vi "DDS Only.vi"() -> ()   [LabVIEW 2013]
doc: "This is the main code used to run experiments in the Cesium laboratory of Mark Saffman. It was written by Martin Lichtman from 2009 to 2012, with DDS drivers written by Alex Gill and Larry Isenhower.\n\nEach hardware section may be enabled and disabled separately. Experiments will finish when all hardware has completed, or when the \"experiment timeout\" is reached, whichever comes first."
uses:
  ExperimentVariables/Variable_Settings.ctl
  DDS_Settings_Cluster.ctl
  DDS Library/Controls/DDS Box Array.ctl
  DDS Library/Controls/DDS Box Cluster.ctl
  DDS Library/Controls/DDS Box Device Reference.ctl
  <vilib>/ni845x/ni845x.llb/ni845xControl.ctl
  DDS Library/Controls/DDS Channel Array.ctl
  DDS Library/Controls/DDS Channel.ctl
  DDS Library/Controls/DDS Channel Parameters.ctl
  DDS Library/Controls/DDS RAM Destination.ctl
  DDS Library/Controls/DDS Profile Array.ctl
  DDS Library/Controls/DDS Profile.ctl
  DDS Library/Controls/DDS RAM Mode.ctl
  DDS Library/Controls/DDS RAM Timestep.ctl
  <vilib>/Utility/error.llb/DialogType.ctl
  config_file_io/all_settings.ctl
  HSDIO/HSDIO_settings.ctl
  <instrlib>/niHSDIO/niHSDIO.llb/niHSDIO_ctl Trigger Script - trigID Values (Ring).ctl
  <instrlib>/niHSDIO/niHSDIO.llb/niHSDIO_ctl Trigger Source Values (Ring).ctl
  <instrlib>/niHSDIO/niHSDIO.llb/niHSDIO_ctl Trigger DigEdge - Edge Values (Ring).ctl
  <instrlib>/niHSDIO/niHSDIO.llb/niHSDIO_ctl Trigger DigLvl - Level Values (Ring).ctl
  DAQmx_pulse_out/settings.ctl
  Camera/Hamamatsu_C9100-13/camera_setup.ctl
  Counter/Counter_Settings_Control.ctl
  filters/filters.ctl
  Analog_output/AO_settings.ctl
  GPIB/HP83623A_RF_Generator/HP83623A_settings.ctl
  PI_piezo/settings.ctl
  PI_piezo/PI_piezo_controller.ctl
  PI_piezo/PI_piezo_channel.ctl
  Camera/Andor/Andor_settings.ctl
  gui/measurement_graph.ctl
  GPIB/RF_Generator_settings_array.ctl
  GPIB/RF_Generator_settings.ctl
  TTL_input/TTL_input_settings.ctl
  Camera/Andor_Luca/Luca_Settings.ctl
  Camera/Andor_Luca/Acquisition_Mode.ctl
  Camera/Andor_Luca/Gain_Mode.ctl
  Aerotech/Aerotech_Settings.ctl
  CONEX-CC/Conex-CC Settings.ctl
  <vilib>/Utility/file.llb/Read From Spreadsheet File (string).vi
  GPIB/HP8662A_RF_Generator/HP8662A_RF_Generator.lvclass
  Camera/Andor_Luca/Andor_Luca.lvclass
  TTL_input/TTL_input.lvclass
  GPIB/GPIB.lvclass
  GPIB/HP83623A_RF_Generator/HP83623A_RF_Generator.lvclass
  Analog_output/Analog_Output.lvclass
  Counter/Counter.lvclass
  Camera/Hamamatsu_C9100-13/Hamamatsu_C9100-13.lvclass
  DDS Library/DDS.lvlib
  DAQmx_pulse_out/DAQmx_pulse_out.lvclass
  HSDIO/HSDIO.lvclass
  ExperimentVariables/ExperimentVariables.lvclass
  Aerotech/Aerotech.lvclass
  CONEX-CC/CONEX-CC.lvclass
panel:
  in  "Save Settings":bool
  in  "Load Settings":bool
  in  "Quit Program":bool=TRUE
  in  "Tab Control":enum32{"Experiment Variables", "DDS"}(tab)=enum."DDS"
  in  "Variable Actions":T1
  in  "Variable Settings":T2={"Measurements per Iteration"=5, "Local Data Path"=path "D:/Hybrid Experiment/Data", "Experiment description suffix for filename (no spaces please)"="TOF_SingleStage", "Network Data Path"=path "Z:/Public/Hybrid/Data/Measurements", "Copy data to network"=TRUE, "Measurement Timeout (ms)"=60000, "Independent Variables"=[{"Description"="MOT Load", "Name (a,a0...a9)"="m", "min"=2000.0, "max"=3000.0, "# steps"=1}, {"Description"="PGC Duration", "Name (a,a0...a9)"="p", "min"=10.0, "max"=10.0, "# steps"=1}, {"Description"="TOF", "Name (a,a0...a9)"="t0", "min"=5.0, "max"=25.0, "# steps"=5}, {"Description"="Exposure", "Name (a,a0...a9)"="e", "min"=0.0, "max"=0.0, "# steps"=1}, {"Description"="Image Pulse", "Name (a,a0...a9)"="i", "min"=1.0, "max"=20.0, "# steps"=1}, {"Description"="ODT Delay", "Name (a,a0...a9)"="d", "min"=0.0, "max"=10.0, "# steps"=1}, {"Description"="Optional ODT on after TOF", "Name (a,a0...a9)"="o", "min"=1.0, "max"=20.0, "# steps"=1}, {"Description"="Depump after PGC", "Name (a,a0...a9)"="r", "min"=0.0, "max"=6.0, "# steps"=1}, {"Description"="Repump In Imaging?", "Name (a,a0...a9)"="i1", "min"=1.0, "max"=1.0, "# steps"=1}, {"Description"="Resonant Blow Away", "Name (a,a0...a9)"="b", "min"=0.0, "max"=0.3, "# steps"=1}, {"Description"="ODT Hold Time", "Name (a,a0...a9)"="h", "min"=0.0, "max"=300.0, "# steps"=1}, {"Description"="HP PGC Stage 1 Duration ", "Name (a,a0...a9)"="m1", "min"=0.0, "max"=20.0, "# steps"=1}, {"Description"="Recapture Time", "Name (a,a0...a9)"="r1", "min"=0.0, "max"=0.0, "# steps"=1}, {"Description"="Trap Turn On Time", "Name (a,a0...a9)"="s", "min"=0.0, "max"=20.0, "# steps"=1}], "Dependent Variables"=[{"Description"="Gamma D1 (MHz)", "Name (a,a0...a9)"="g1", "Equation"="4.5612", "Result"=4.5612}, {"Description"="Gamma D2 (MHz)", "Name (a,a0...a9)"="g2", "Equation"="5.2227", "Result"=5.2227}, {"Description"="MOT Power (mW)", "Name (a,a0...a9)"="p0", "Equation"="18.0", "Result"=18.0}, {"Description"="MOT Detuning (MHz)", "Name (a,a0...a9)"="d0", "Equation"="126.2", "Result"=126.2}, {"Description"="MOT Beam Waist (mm)", "Name (a,a0...a9)"="w0", "Equation"="2.3", "Result"=2.3}, {"Description"="PGC_0 Power (mW)", "Name (a,a0...a9)"="h3", "Equation"="2", "Result"=2.0}, {"Description"="PGC_0 Frequency (MHz)", "Name (a,a0...a9)"="h4", "Equation"="117", "Result"=117.0}, {"Description"="PGC Power (mW)", "Name (a,a0...a9)"="p1", "Equation"="5", "Result"=5.0}, {"Description"="PGC Detuning (MHz)", "Name (a,a0...a9)"="d1", "Equation"="-7.7*g2", "Result"=-40.21479}, {"Description"="Imaging Power (mW)", "Name (a,a0...a9)"="p2", "Equation"="18", "Result"=18.0}, {"Description"="Imaging Frequency (MHz) ", "Name (a,a0...a9)"="d2", "Equation"="126.2", "Result"=126.2}, {"Description"="Repump Power (mW)", "Name (a,a0...a9)"="p3", "Equation"="3.4", "Result"=3.4}, {"Description"="Repump Waist (mm)", "Name (a,a0...a9)"="w3", "Equation"="2.3", "Result"=2.3}, {"Description"="OP Power (mW)", "Name (a,a0...a9)"="p4", "Equation"="0", "Result"=0.0}, {"Description"="OP Detuning (MHz)", "Name (a,a0...a9)"="d4", "Equation"="0", "Result"=0.0}, {"Description"="OP Waist (mm)", "Name (a,a0...a9)"="w4", "Equation"="0", "Result"=0.0}, {"Description"="Raman Power (mW)", "Name (a,a0...a9)"="p5", "Equation"="0", "Result"=0.0}, {"Description"="Raman Detuning (MHz)", "Name (a,a0...a9)"="d5", "Equation"="0", "Result"=0.0}, {"Description"="Raman Waist (mm)", "Name (a,a0...a9)"="w5", "Equation"="0", "Result"=0.0}, {"Description"="685nm Power (mW)", "Name (a,a0...a9)"="p6", "Equation"="0", "Result"=0.0}, {"Description"="685nm Detuning (MHz)", "Name (a,a0...a9)"="d6", "Equation"="0", "Result"=0.0}, {"Description"="685nm Waist (um)", "Name (a,a0...a9)"="w6", "Equation"="0", "Result"=0.0}, {"Description"="595nm Power (mW)", "Name (a,a0...a9)"="p7", "Equation"="0", "Result"=0.0}, {"Description"="595nm Detuning (MHz)", "Name (a,a0...a9)"="d7", "Equation"="0", "Result"=0.0}, {"Description"="595nm Waist (mm)", "Name (a,a0...a9)"="w7", "Equation"="0", "Result"=0.0}, {"Description"="935nm Power (mW)", "Name (a,a0...a9)"="p8", "Equation"="246", "Result"=246.0}, {"Description"="935nm Waist (mm)", "Name (a,a0...a9)"="w8", "Equation"="0.011", "Result"=0.011}, {"Description"="935 VVA Voltage (V)", "Name (a,a0...a9)"="v8", "Equation"="5.65", "Result"=5.65}, {"Description"="802nm Power (mW)", "Name (a,a0...a9)"="p9", "Equation"="0", "Result"=0.0}, {"Description"="802nm Wiast (mm)", "Name (a,a0...a9)"="w9", "Equation"="0", "Result"=0.0}, {"Description"="X Initial Position (mm)", "Name (a,a0...a9)"="x0", "Equation"="30.5", "Result"=30.5}, {"Description"="X Final Position (mm)", "Name (a,a0...a9)"="x1", "Equation"="35.5", "Result"=35.5}, {"Description"="X Max. Velocity (m/s)", "Name (a,a0...a9)"="a0", "Equation"="100", "Result"=100.0}, {"Description"="X Max. Accn. (m/s^2)", "Name (a,a0...a9)"="v0", "Equation"="2500", "Result"=2500.0}, {"Description"="MOT Shutter Open Delay (ms)", "Name (a,a0...a9)"="o0", "Equation"="2.96", "Result"=2.96}, {"Description"="MOT Shutter Close Delay (ms)", "Name (a,a0...a9)"="c0", "Equation"="3.32", "Result"=3.32}], "Run Test Mode"=FALSE} {"Independent Variables"."# steps" min=1 step=1; "Measurements per Iteration" min=1 step=1}
  in  "DDS Settings":T3={"Enable DDS"=TRUE, "Array of DDS Boxes"=[{"DDS box device reference"={"NI USB-8451 device reference"="DDS_Box4", "DIO port"=0, "Serial Clock Rate [kHz]"=1000}, "Array of DDS Channels (4)"=[{"Power"=FALSE, "Channel Parameters"={"Ref Clock Rate [MHz]"=1000.0, "Full Scale Output\nPower [dBm]"=0.0}, "RAM Enable"=FALSE, "RAM Dest Type"=enum."Frequency", "RAM Default"={"Frequency [MHz]"="80", "Amplitude [dBm]"="0", "Phase Offset [rad]"="0"}, "Array of DDS Profiles (8)"=[], "Description"=""}, {"Power"=FALSE, "Channel Parameters"={"Ref Clock Rate [MHz]"=1000.0, "Full Scale Output\nPower [dBm]"=0.0}, "RAM Enable"=FALSE, "RAM Dest Type"=enum."Frequency", "RAM Default"={"Frequency [MHz]"="80", "Amplitude [dBm]"="0", "Phase Offset [rad]"="0"}, "Array of DDS Profiles (8)"=[], "Description"=""}, {"Power"=FALSE, "Channel Parameters"={"Ref Clock Rate [MHz]"=1000.0, "Full Scale Output\nPower [dBm]"=0.0}, "RAM Enable"=FALSE, "RAM Dest Type"=enum."Frequency", "RAM Default"={"Frequency [MHz]"="80", "Amplitude [dBm]"="0", "Phase Offset [rad]"="0"}, "Array of DDS Profiles (8)"=[], "Description"=""}, {"Power"=TRUE, "Channel Parameters"={"Ref Clock Rate [MHz]"=1000.0, "Full Scale Output\nPower [dBm]"=0.0}, "RAM Enable"=TRUE, "RAM Dest Type"=enum."Frequency", "RAM Default"={"Frequency [MHz]"="190", "Amplitude [dBm]"="0", "Phase Offset [rad]"="0"}, "Array of DDS Profiles (8)"=[{"Single Tone"={"Frequency [MHz]"="202.5", "Amplitude [dBm]"="0", "Phase Offset [rad]"="0"}, "RAM Mode "=enum."Continuous Bidirectional Ramp", "Zero-crossing"=FALSE, "No Dwell High"=FALSE, "Function/Static"=FALSE, "RAM Function Settings"=["", "", "", "100"], "RAM Static Array"=[[190.0, 200.0]], "Description"="", "Time Step (us)"=0.0}], "Description"=""}], "Enable"=TRUE, "Description"=""}]} {"Array of DDS Boxes"."Array of DDS Channels (4)"."Channel Parameters"."Ref Clock Rate [MHz]" min=0.0}
  in  "DDS Actions":T16
  out "DDS Initialized":bool=TRUE
  in  "box #":i32=2 min=0 step=1
  out "CFR3":u8[][](array[numeric])=[[31, 63, 192, 0], [31, 63, 192, 0], [31, 63, 192, 0], [31, 63, 192, 0]]
  out "CFR2":u8[][](array[numeric])=[[1, 64, 8, 32], [1, 64, 8, 32], [1, 64, 8, 32], [1, 64, 8, 32]]
  out "CFR1":u8[][](array[numeric])=[[0, 0, 0, 2], [0, 0, 0, 2], [0, 0, 0, 2], [0, 0, 0, 242]]
  in  "Check DDS":bool
  # "Parameters will be evaluated once at the beginning of the experiment from top to bottom, \nso any parameter may depend on all those above it.\nVariables will be evaluated each iteration.\nParameters and Variables may be used in various other experiment settings, as noted.\nSee LabView Help -> Formula Node and Expression Node Functions for a list of available functions."
  # "f/f/A"
  # "Mag"
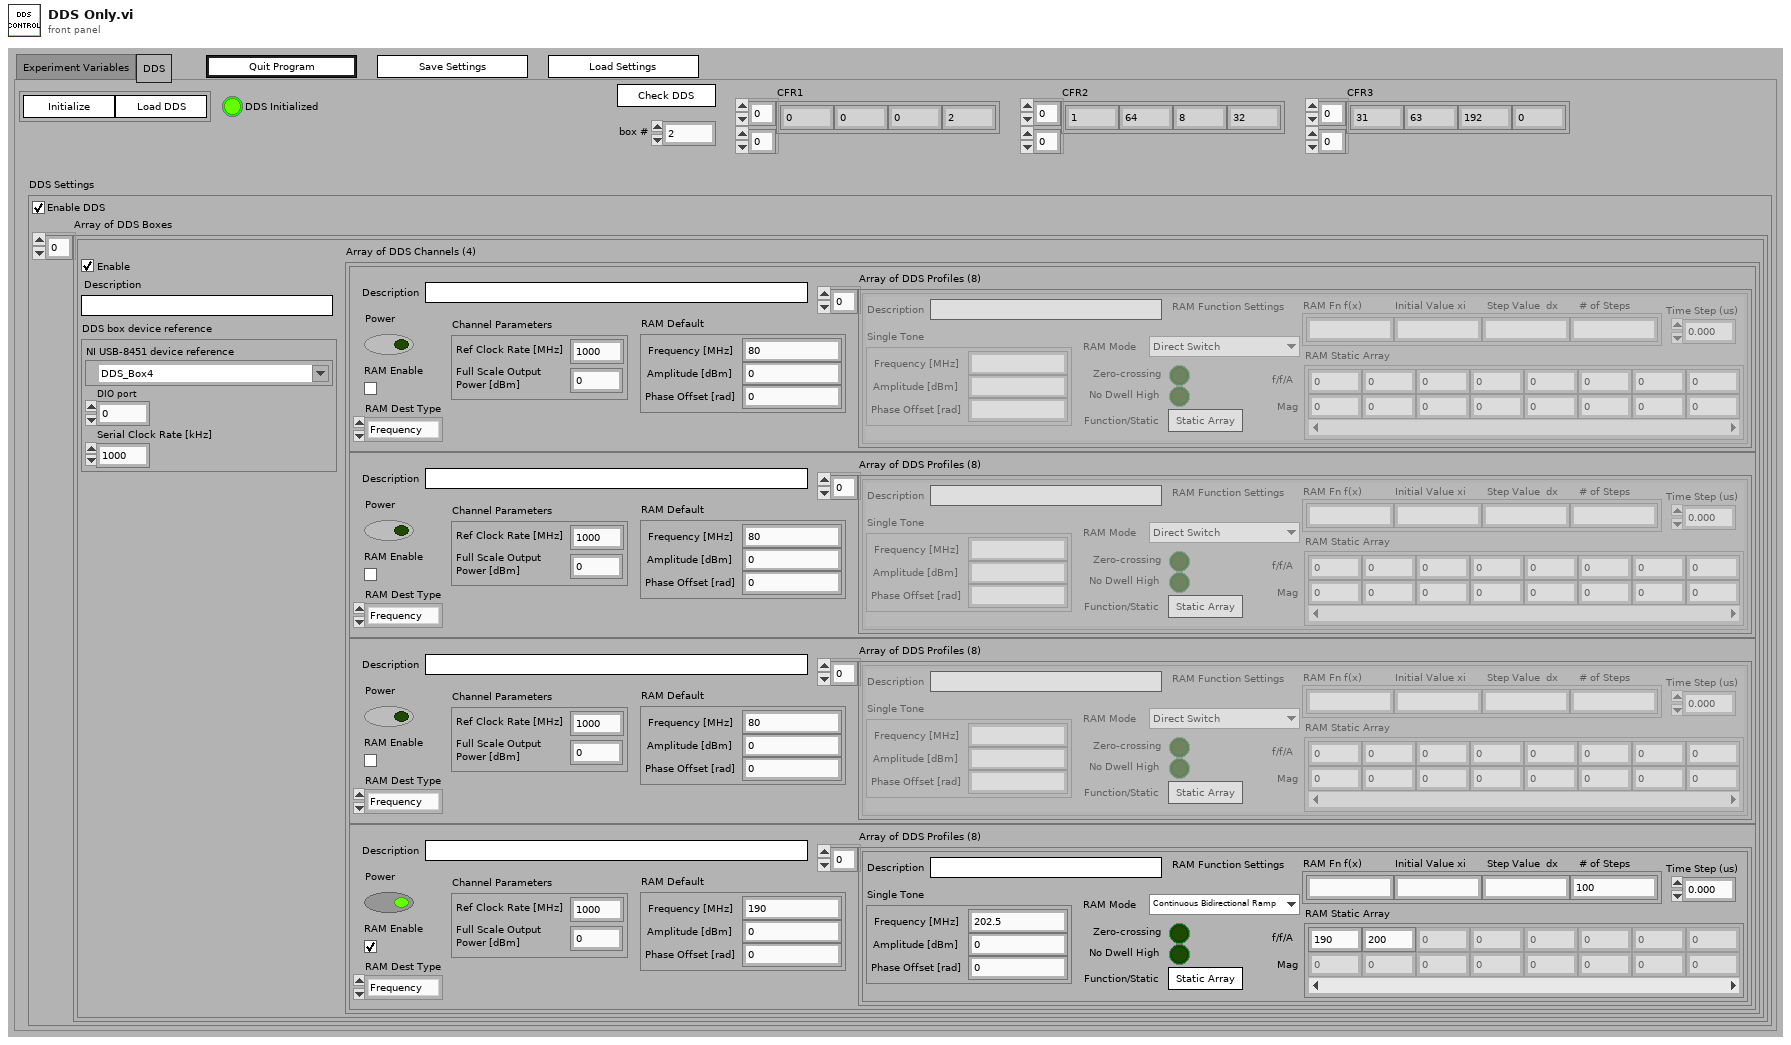
[diagram p1: front panel]
types:
  T1 = cluster{"Load Independents":bool, "Save Independents":bool, "Load Dependents":bool, "Save Dependents":bool, "Evaluate Dependents":bool, "Clear Log":bool, "Save Log":bool}
  T2 = typedef "ExperimentVariables.lvclass/Variable_Settings.ctl" = cluster{"Measurements per Iteration":i32, "Local Data Path":path, "Experiment description suffix for filename (no spaces please)":string, "Network Data Path":path, "Copy data to network":bool, "Measurement Timeout (ms)":u32, "Independent Variables":cluster{"Description":string, "Name (a,a0...a9)":string, "min":dbl, "max":dbl, "# steps":u32}[], "Dependent Variables":cluster{"Description":string, "Name (a,a0...a9)":string, "Equation":string, "Result":dbl}[], "Run Test Mode":bool}
  T3 = typedef "DDS_Settings_Cluster.ctl" = cluster{"Enable DDS":bool, "Array of DDS Boxes":T4}
  T4 = typedef "DDS.lvlib/DDS Box Array.ctl" = T5[]
  T5 = typedef "DDS.lvlib/DDS Box Cluster.ctl" = cluster{"DDS box device reference":T6, "Array of DDS Channels (4)":T8, "Enable":bool, "Description":string}
  T6 = typedef "DDS.lvlib/DDS Box Device Reference.ctl" = cluster{"NI USB-8451 device reference":T7, "DIO port":u8, "Serial Clock Rate [kHz]":u16}
  T7 = typedef "ni845xControl.ctl" = refnum<k21>
  T8 = typedef "DDS.lvlib/DDS Channel Array.ctl" = T9[]
  T9 = typedef "DDS.lvlib/DDS Channel.ctl" = cluster{"Power":bool, "Channel Parameters":T10, "RAM Enable":bool, "RAM Dest Type":T11, "RAM Default":cluster{"Frequency [MHz]":string, "Amplitude [dBm]":string, "Phase Offset [rad]":string}, "Array of DDS Profiles (8)":T12, "Description":string}
  T10 = typedef "DDS.lvlib/DDS Channel Parameters.ctl" = cluster{"Ref Clock Rate [MHz]":dbl, "Full Scale Output\nPower [dBm]":dbl}
  T11 = typedef "DDS.lvlib/DDS RAM Destination.ctl" = enum16{"Frequency", "Phase", "Amplitude", "Polar"}
  T12 = typedef "DDS.lvlib/DDS Profile Array.ctl" = T13[]
  T13 = typedef "DDS.lvlib/DDS Profile.ctl" = cluster{"Single Tone":cluster{"Frequency [MHz]":string, "Amplitude [dBm]":string, "Phase Offset [rad]":string}, "RAM Mode ":T14, "Zero-crossing":bool, "No Dwell High":bool, "Function/Static":bool, "RAM Function Settings":string[], "RAM Static Array":dbl[][], "Description":string, "Time Step (us)":T15}
  T14 = typedef "DDS.lvlib/DDS RAM mode.ctl" = enum16{"Direct Switch", "Ramp Up", "Bidirectional Ramp", "Continuous Bidirectional Ramp", "Continuous Recirculate", "Direct Switch 2", "Direct Switch 3", "Direct Switch 4"}
  T15 = typedef "DDS.lvlib/DDS RAM Timestep.ctl" = dbl
  T16 = cluster{"Initialize DDS Boxes":bool, "Load DDS":bool}
  T17 = typedef "DialogType.ctl" = u16
  T18 = cluster{"Description":string, "Name (a,a0...a9)":string, "min":dbl, "max":dbl, "# steps":u32}
  T19 = cluster{"Description":string, "Name (a,a0...a9)":string, "Equation":string, "Result":dbl}
  T20 = typedef "all_settings.ctl" = cluster{"Variable Settings":T2, "HSDIO Settings":T21, "DAQmx Pulse Settings":T26, "DDS Settings":T3, "Hamamatsu settings":T27, "Counter Settings":T28, "Filter Cluster":T29, "Analog Output Parameters":T30, "Notes":string, "HP83623A Generator Settings Array":T31, "Iteration Graph Settings":cluster{"Plot Regions":string, "Plot Shots":string}, "PI Piezo Settings":T32, "Andor settings":T35, "Measurement Chart Settings":T36, "HP8662A Synthesized Signal Generator Array":T37, "HP83712B Synthesized CW Generator Array":T37, "TTL input":T39, "Luca Settings":T40, "AFG3102 Frequency Control (kHz only)":T38, "Aerotech Settings":T43, "CONEX-CC Settings":T44}
  T21 = typedef "HSDIO.lvclass/HSDIO_settings.ctl" = cluster{"Enable HSDIO Pulses":bool, "Resource Name":refnum<k15>, "Clock Rate":dbl, "units/sec (ms=1000)":dbl, "Array of Script Triggers":cluster{"trigger id (script trigger 0)":T22, "source (PFI 0)":T23, "Trigger Type":enum32{"Edge", "Level"}, "edge":T24, "level":T25}[], "Channels Control":string[][], "Pulse Generation Script":string, "Directory to look for waveform files":path, "Start Trigger":cluster{"Wait for start trigger?":bool, "source (PFI 0)":T23, "edge (rising)":T24}, "Hardware alignment quantum\n(in samples)":u16, "Use file script":bool, "Base path for script":path, "filename for script":string}
  T22 = typedef "niHSDIO_ctl Trigger Script - trigID Values (Ring).ctl" = string
  T23 = typedef "niHSDIO_ctl Trigger Source Values (Ring).ctl" = string
  T24 = typedef "niHSDIO_ctl Trigger DigEdge - Edge Values (Ring).ctl" = i32
  T25 = typedef "niHSDIO_ctl Trigger DigLvl - Level Values (Ring).ctl" = i32
  T26 = typedef "DAQmx_pulse_out.lvclass/settings.ctl" = cluster{"Enable DAQmx Pulses":bool, "DAQmx Physical Channels":tag, "Clock Rate":dbl, "units/sec (ms=1000)":dbl, "Start Trigger":cluster{"Wait for start trigger?":bool, "source":tag, "edge":i32}, "Timing Sequence Control":string[][]}
  T27 = typedef "Hamamatsu_C9100-13.lvclass/camera_setup.ctl" = cluster{"Analog Gain (0-5)":u8, "Frame Grabber acquisition region\n(left, top, right, bottom)":i32[], "Exposure Time":dbl, "EM Gain (0-255)":u8, "Trigger Polarity":string, "External Trigger Mode":string, "Scan Speed":string, "External Trigger Source":string, "Scan Mode":string, "Super Pixel Binning\n(if enabled in Scan Mode)":string, "Camera Sub-array acquisition region\n(if enabled in scan mode)":cluster{"Left":u16, "Top":u16, "Width":u16, "Height":u16}, "Use camera?":bool, "# image buffers":i32, "Regions of Interest (Left, Top, Right, Bottom)":i32[][], "Background Regions (Left, Top, Right, Bottom)":i32[][], "shots per measurement":i32, "Photoelectron Scaling":dbl, "Low Light\nSensitivity":string, "Save as TIF?":bool, "Save as Raw .dat?":bool, "Cooling":string, "Fan":string}
  T28 = typedef "Counter.lvclass/Counter_Settings_Control.ctl" = cluster{"Enable Counters":bool, "Array of Counter Settings":cluster{"Counter Channel":tag, "Time-Bin Clock Channel":tag, "Binwidth (ms)":dbl}[], "#Bins to drop":i32, "Total Counts Active Bins":i32[][], "Histogram":cluster{"Active Bins (Bin i:j)":i32[][], "Histogram?":bool, "Accumulate?":bool}}
  T29 = typedef "filters.ctl" = cluster{"Counter Filter thresholds":u32[][], "Data Filters\nROI Minimum Thresholds":u64[][]}
  T30 = typedef "Analog_Output.lvclass/AO_settings.ctl" = cluster{"Enable Analog Out?":bool, "Physical Channel":tag, "Minimum Value":dbl, "Maximum Value":dbl, "Samples per second":string, "Total AO Time (seconds)":string, "Analog Output Equations for each Channel":string[], "Start Trigger":cluster{"Wait for start trigger?":bool, "source":tag, "edge":i32}, "AO Channel List":string[]}
  T31 = typedef "HP83623A_RF_Generator.lvclass/HP83623A_settings.ctl" = cluster{"Frequency (Hz)":string, "Power (dBm)":string, "Enabled":bool, "initialized":bool, "RF Output On/Off":bool, "External Trigger?":bool, "VISA Session":refnum<visa-resource-name>, "Generator Name":string}[]
  T32 = typedef "settings.ctl" = cluster{"Enable":bool, "Array of Piezo Controllers":T33[]}
  T33 = typedef "PI_piezo_controller.ctl" = cluster{"Enable":bool, "Serial No.":string, "Array of Piezo Channels":T34[]}
  T34 = typedef "PI_piezo_channel.ctl" = cluster{"Servo":bool, "Set Position":string, "Drift Compensation":bool}
  T35 = typedef "Andor_settings.ctl" = cluster{"Andor Path":path, "Copy any Andor files":bool, "Wait time before copying Andor files (ms)":u16}
  T36 = typedef "measurement_graph.ctl" = cluster{"Which regions to plot (comma separated)":string, "Which shot to plot":u8}
  T37 = typedef "GPIB.lvclass/RF_Generator_settings_array.ctl" = T38[]
  T38 = typedef "GPIB.lvclass/RF_Generator_settings.ctl" = cluster{"Enable":bool, "Description":string, "GPIB channel #":u8, "Frequency (MHz)":string, "Power (dBm)":string}
  T39 = typedef "TTL_input.lvclass/TTL_input_settings.ctl" = cluster{"Enable":bool, "lines":tag}
  T40 = typedef "Andor_Luca.lvclass/Luca_Settings.ctl" = cluster{"Active Pixels (Left,Right,Top,Bottom)":i32[], "Pixel Binning":string, "Use camera?":bool, "Regions of Interest (Left, Top, Right, Bottom)":i32[][], "Background Regions (Left, Top, Right, Bottom)":i32[][], "Photoelectron Scaling":dbl, "Save as TIF":bool, "Save as Raw .dat":bool, "Acquisition Mode":T41, "Gain Mode":T42, "Trigger Mode":string, "Fan Mode":string, "Advanced EMgain":bool, "EMCCD Gain (0-200/1000)":u32, "Exposure (s)":sgl, "#Kinetics":i32, "Hbin":i32, "Vbin":i32, "#H":i32, "#V":i32, "BG Subtraction":bool}
  T41 = typedef "Acquisition_Mode.ctl" = string
  T42 = typedef "Gain_Mode.ctl" = string
  T43 = typedef "Aerotech.lvclass/Aerotech_Settings.ctl" = cluster{"Enable":bool, "DGLOBAL Array":string[][], "DGlobal_Update":bool, "IGLOBAL Array":string[][], "IGlobal_Update":bool}
  T44 = typedef "CONEX-CC.lvclass/Conex-CC Settings.ctl" = cluster{"Enabled?":bool, "Set Position":string, "Velocity (mm/s)":dbl, "ModVel?":bool}
  T45 = cluster{"Description":string, "Name (a,a0...a9)":string, "min":dbl, "max":dbl, "# steps":u32}[]
  T46 = cluster{"Description":string, "Name (a,a0...a9)":string, "Equation":string, "Result":dbl}[]
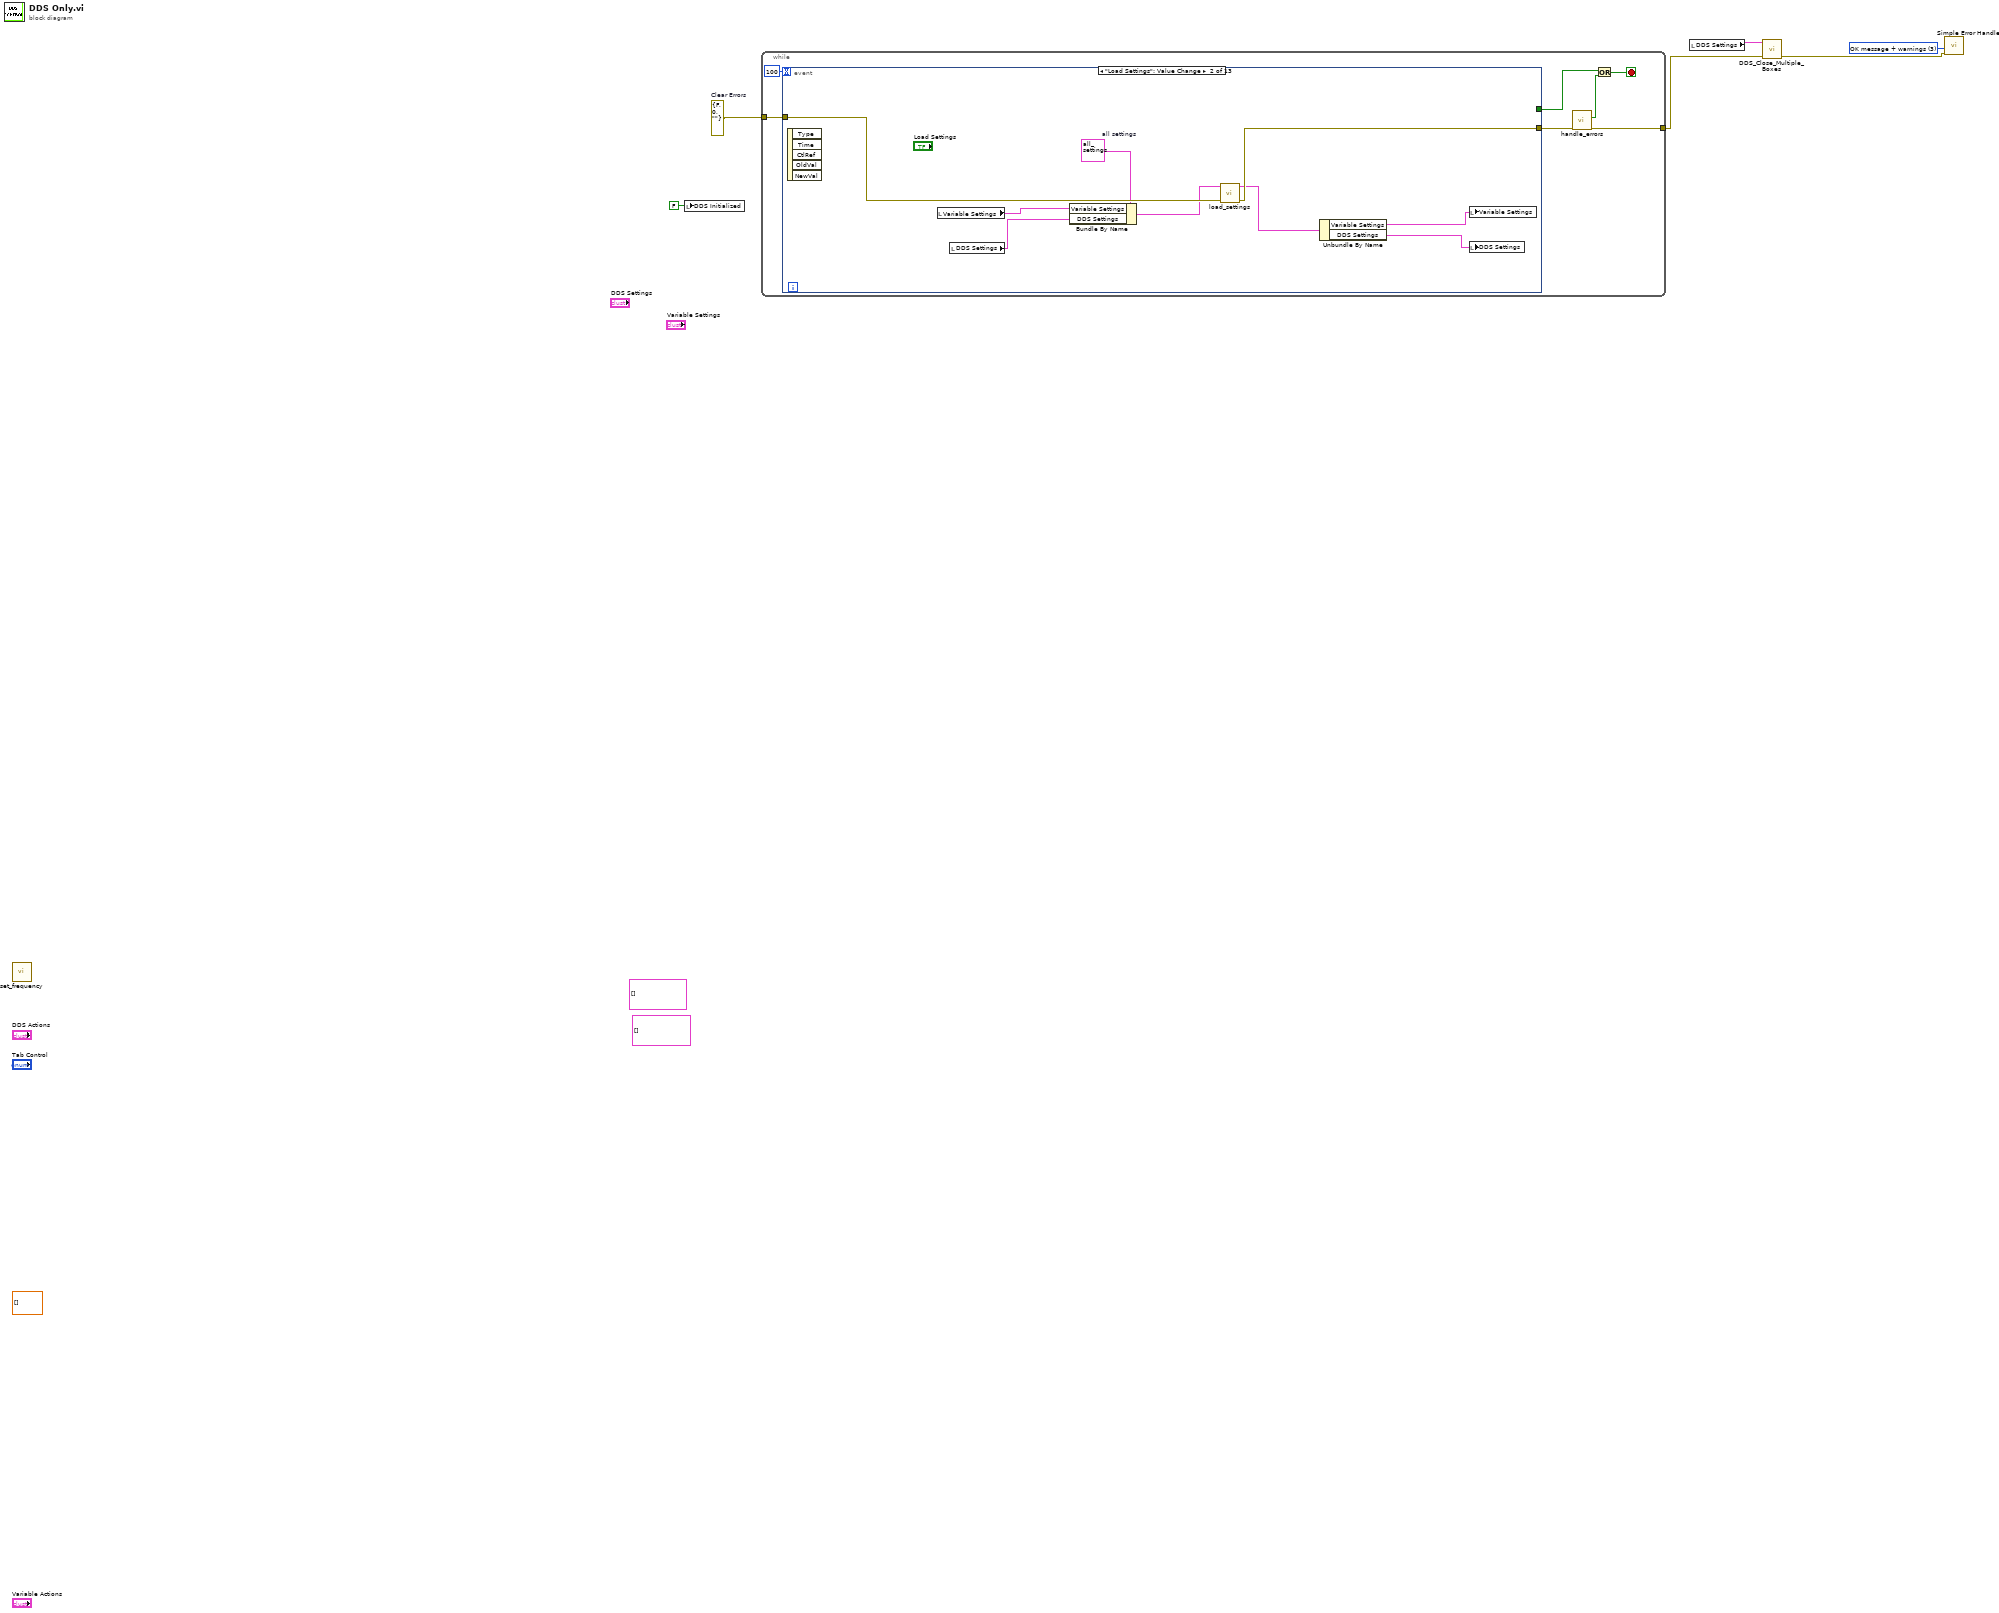
[diagram p0: block diagram]
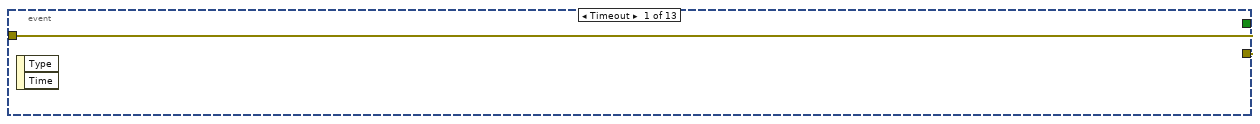
[diagram p2: hidden frame]
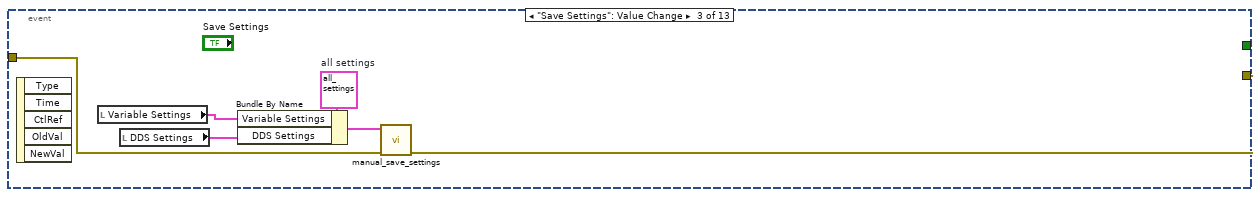
[diagram p3: hidden frame]
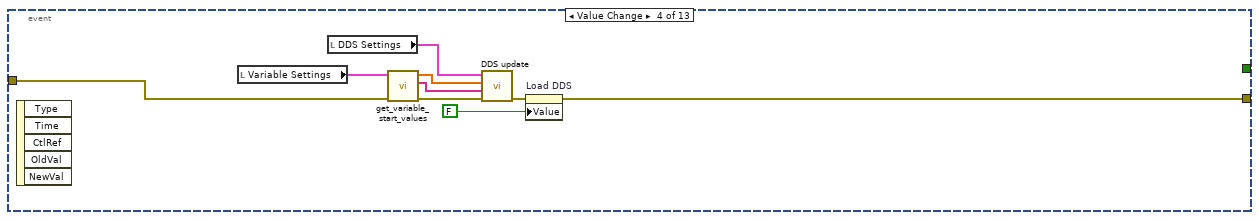
[diagram p4: hidden frame]
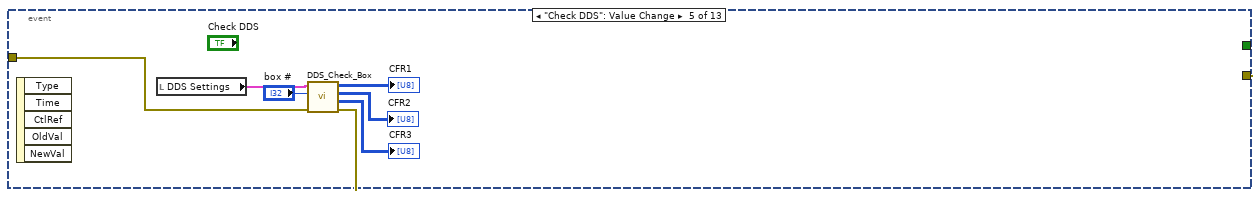
[diagram p5: hidden frame]
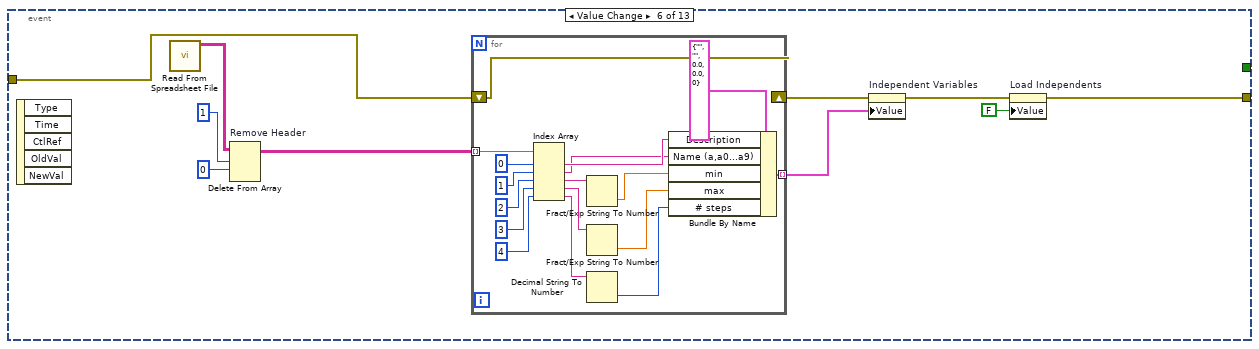
[diagram p6: hidden frame]
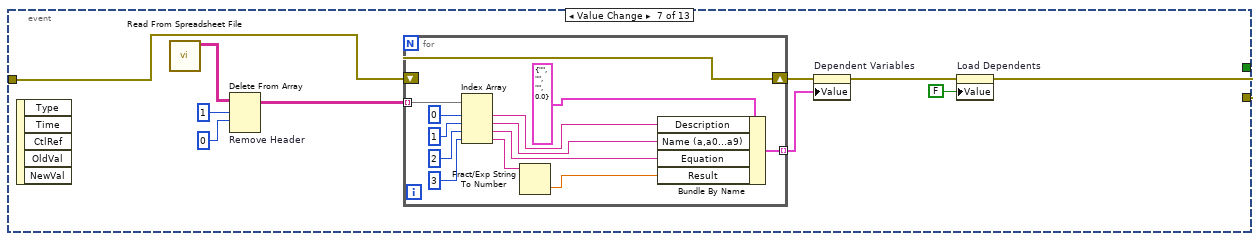
[diagram p7: hidden frame]
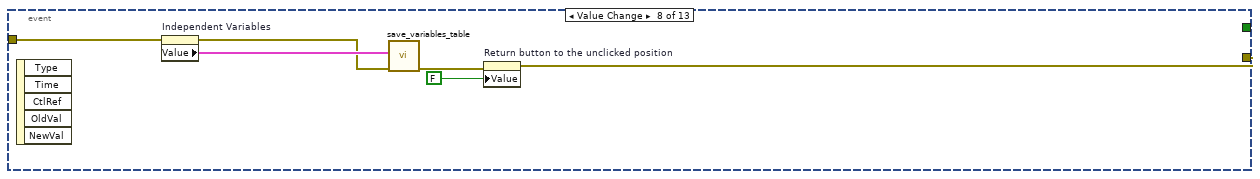
[diagram p8: hidden frame]
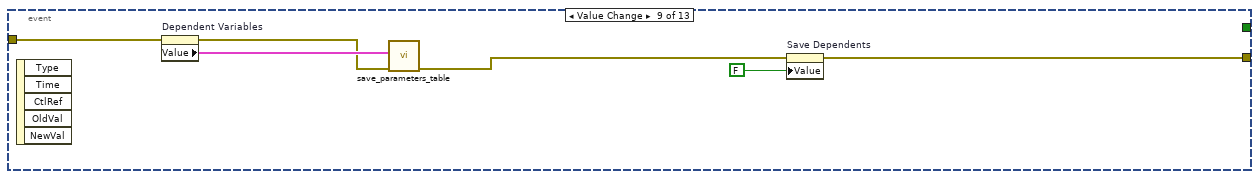
[diagram p9: hidden frame]
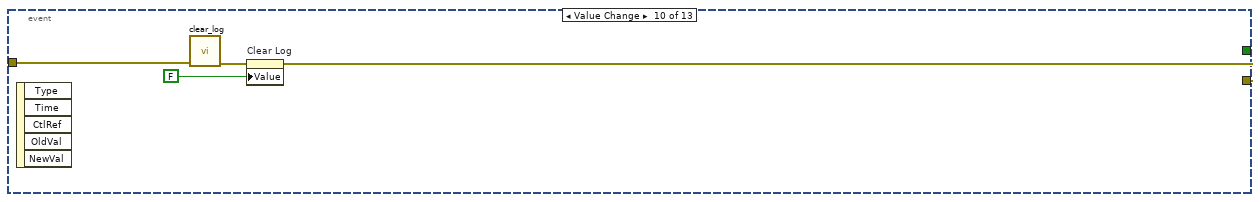
[diagram p10: hidden frame]
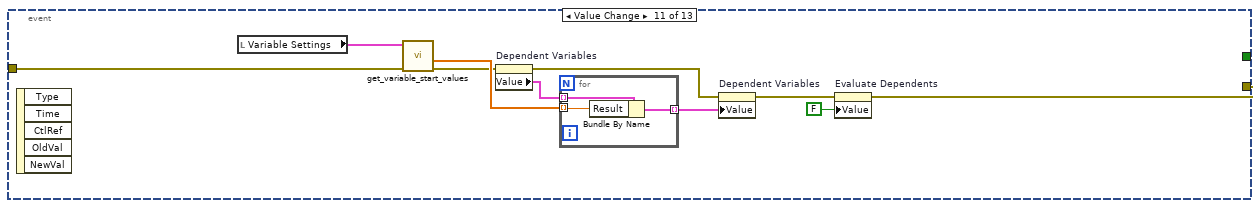
[diagram p11: hidden frame]
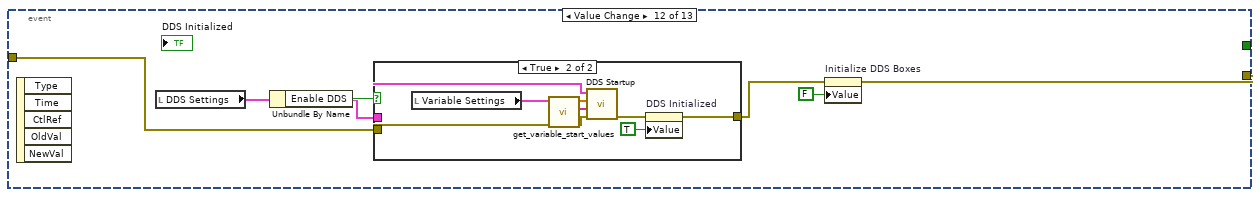
[diagram p12: hidden frame]
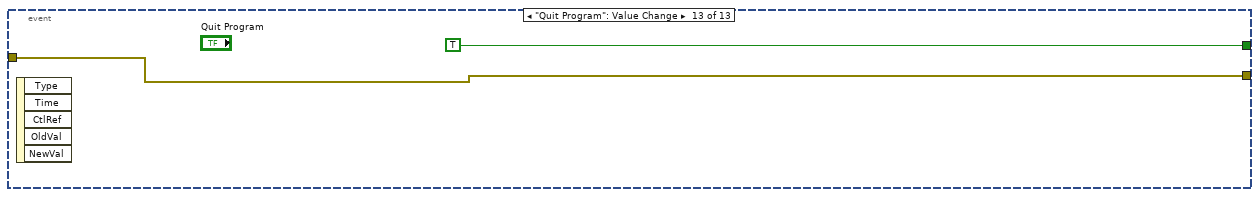
[diagram p14: hidden frame]
diagram:
  (unwired) cluster{"Iteration Total 2":i32[][]}[] [] ("All Iteration Histogram Data")
  (unwired) cluster{"Iteration Total 2":dbl[][]}[] [] ("All Iteration Average Data")
  (unwired) dbl[][] [] ("Iteration Graph")
  w6 = T17 3 items=["no dialog", "OK message", "continue or stop message", "OK message + warnings", "continue/stop + warnings"] ("type of dialog (OK msg:1)")
  w2 = errorcluster {"status"=FALSE, "code"=0, "source"=""}  # Clear Errors
  n1 = call "set_frequency.vi"() -> ()  [unwired: 11 in, 1 out]
  n2 = local write "DDS Initialized"(FALSE ("DDS Initialized")) -> ()
  n3 = while {
    tunnel: w2 -> [w13]
    tunnel: [w9] -> w5
    stop <- w12 stop-if-true
    n4 = event shown="[1] \"Load Settings\": Value Change" {
      selector: _ -> [_ _ _ _ _ _ _ _ _ _ _ _ _]
      dyn-events: _ -> [_ _ _ _ _ _ _ _ _ _ _ _ _]
      timeout: 100 -> [_ _ _ _ _ _ _ _ _ _ _ _ _]
      tunnel: w13 -> [w14 w23 w26 w31 w45 w50 w80 w99 w105 w109 w115 w130 w141]
      tunnel: [w14 w22 w25 w34 w44 w55 w82 w100 w107 w110 w121 w127 w141] -> w11
      tunnel: [_ _ _ _ _ _ _ _ _ _ _ _ TRUE] -> w10
      event Timeout {
        n5 = event-data() -> ()  [unwired: 1 in, 2 out]
      }
      event "Load Settings": Value Change {
        w20 = T20 {"Variable Settings"={"Measurements per Iteration"=0, "Local Data Path"=path "", "Experiment description suffix for filename (no spaces please)"="", "Network Data Path"=path "", "Copy data to network"=FALSE, "Measurement Timeout (ms)"=0, "Independent Variables"=[], "Dependent Variables"=[], "Run Test Mode"=FALSE}, "HSDIO Settings"={"Enable HSDIO Pulses"=FALSE, "Resource Name"="", "Clock Rate"=0.0, "units/sec (ms=1000)"=0.0, "Array of Script Triggers"=[], "Channels Control"=[], "Pulse Generation Script"="", "Directory to look for waveform files"=path "", "Start Trigger"={"Wait for start trigger?"=FALSE, "source (PFI 0)"="", "edge (rising)"=0}, "Hardware alignment quantum\n(in samples)"=0, "Use file script"=FALSE, "Base path for script"=path "", "filename for script"=""}, "DAQmx Pulse Settings"={"Enable DAQmx Pulses"=FALSE, "DAQmx Physical Channels"="", "Clock Rate"=0.0, "units/sec (ms=1000)"=0.0, "Start Trigger"={"Wait for start trigger?"=FALSE, "source"="", "edge"=0}, "Timing Sequence Control"=[]}, "DDS Settings"={"Enable DDS"=FALSE, "Array of DDS Boxes"=[]}, "Hamamatsu settings"={"Analog Gain (0-5)"=0, "Frame Grabber acquisition region\n(left, top, right, bottom)"=[], "Exposure Time"=0.0, "EM Gain (0-255)"=0, "Trigger Polarity"="", "External Trigger Mode"="", "Scan Speed"="", "External Trigger Source"="", "Scan Mode"="", "Super Pixel Binning\n(if enabled in Scan Mode)"="", "Camera Sub-array acquisition region\n(if enabled in scan mode)"={"Left"=0, "Top"=0, "Width"=0, "Height"=0}, "Use camera?"=FALSE, "# image buffers"=0, "Regions of Interest (Left, Top, Right, Bottom)"=[], "Background Regions (Left, Top, Right, Bottom)"=[], "shots per measurement"=0, "Photoelectron Scaling"=0.0, "Low Light\nSensitivity"="", "Save as TIF?"=FALSE, "Save as Raw .dat?"=FALSE, "Cooling"="", "Fan"=""}, "Counter Settings"={"Enable Counters"=FALSE, "Array of Counter Settings"=[], "#Bins to drop"=0, "Total Counts Active Bins"=[], "Histogram"={"Active Bins (Bin i:j)"=[], "Histogram?"=FALSE, "Accumulate?"=FALSE}}, "Filter Cluster"={"Counter Filter thresholds"=[], "Data Filters\nROI Minimum Thresholds"=[]}, "Analog Output Parameters"={"Enable Analog Out?"=FALSE, "Physical Channel"="", "Minimum Value"=0.0, "Maximum Value"=0.0, "Samples per second"="", "Total AO Time (seconds)"="", "Analog Output Equations for each Channel"=[], "Start Trigger"={"Wait for start trigger?"=FALSE, "source"="", "edge"=0}, "AO Channel List"=[]}, "Notes"="", "HP83623A Generator Settings Array"=[], "Iteration Graph Settings"={"Plot Regions"="", "Plot Shots"=""}, "PI Piezo Settings"={"Enable"=FALSE, "Array of Piezo Controllers"=[]}, "Andor settings"={"Andor Path"=path "", "Copy any Andor files"=FALSE, "Wait time before copying Andor files (ms)"=0}, "Measurement Chart Settings"={"Which regions to plot (comma separated)"="", "Which shot to plot"=0}, "HP8662A Synthesized Signal Generator Array"=[], "HP83712B Synthesized CW Generator Array"=[], "TTL input"={"Enable"=FALSE, "lines"=""}, "Luca Settings"={"Active Pixels (Left,Right,Top,Bottom)"=[], "Pixel Binning"="", "Use camera?"=FALSE, "Regions of Interest (Left, Top, Right, Bottom)"=[], "Background Regions (Left, Top, Right, Bottom)"=[], "Photoelectron Scaling"=0.0, "Save as TIF"=FALSE, "Save as Raw .dat"=FALSE, "Acquisition Mode"="", "Gain Mode"="", "Trigger Mode"="", "Fan Mode"="", "Advanced EMgain"=FALSE, "EMCCD Gain (0-200/1000)"=0, "Exposure (s)"=0.0, "#Kinetics"=0, "Hbin"=0, "Vbin"=0, "#H"=0, "#V"=0, "BG Subtraction"=FALSE}, "AFG3102 Frequency Control (kHz only)"={"Enable"=FALSE, "Description"="", "GPIB channel #"=0, "Frequency (MHz)"="", "Power (dBm)"=""}, "Aerotech Settings"={"Enable"=FALSE, "DGLOBAL Array"=[], "DGlobal_Update"=FALSE, "IGLOBAL Array"=[], "IGlobal_Update"=FALSE}, "CONEX-CC Settings"={"Enabled?"=FALSE, "Set Position"="", "Velocity (mm/s)"=0.0, "ModVel?"=FALSE}}  # all settings
        n6 = event-data() -> ()  [unwired: 1 in, 5 out]
        n7 = local read "Variable Settings"() -> (w19:T2)
        n8 = local read "DDS Settings"() -> (w21:T3)
        n9 = Bundle By Name(cluster=w20, "Variable Settings"=w19, "DDS Settings"=w21) -> (w18:T20)
        n10 = call "load_settings.vi"("error in"=w23, "all settings (in)"=w18) -> ("error out"=w22:errorcluster, "all settings"=w15:T20)  [unwired: 8 in]
        n11 = Unbundle By Name(w15) -> ("Variable Settings"=w17:T2, "DDS Settings"=w16:T3)
        n12 = local write "Variable Settings"(w17) -> ()
        n13 = local write "DDS Settings"(w16) -> ()
      }
      event "Save Settings": Value Change {
        w29 = T20 {"Variable Settings"={"Measurements per Iteration"=0, "Local Data Path"=path "", "Experiment description suffix for filename (no spaces please)"="", "Network Data Path"=path "", "Copy data to network"=FALSE, "Measurement Timeout (ms)"=0, "Independent Variables"=[], "Dependent Variables"=[], "Run Test Mode"=FALSE}, "HSDIO Settings"={"Enable HSDIO Pulses"=FALSE, "Resource Name"="", "Clock Rate"=0.0, "units/sec (ms=1000)"=0.0, "Array of Script Triggers"=[], "Channels Control"=[], "Pulse Generation Script"="", "Directory to look for waveform files"=path "", "Start Trigger"={"Wait for start trigger?"=FALSE, "source (PFI 0)"="", "edge (rising)"=0}, "Hardware alignment quantum\n(in samples)"=0, "Use file script"=FALSE, "Base path for script"=path "", "filename for script"=""}, "DAQmx Pulse Settings"={"Enable DAQmx Pulses"=FALSE, "DAQmx Physical Channels"="", "Clock Rate"=0.0, "units/sec (ms=1000)"=0.0, "Start Trigger"={"Wait for start trigger?"=FALSE, "source"="", "edge"=0}, "Timing Sequence Control"=[]}, "DDS Settings"={"Enable DDS"=FALSE, "Array of DDS Boxes"=[]}, "Hamamatsu settings"={"Analog Gain (0-5)"=0, "Frame Grabber acquisition region\n(left, top, right, bottom)"=[], "Exposure Time"=0.0, "EM Gain (0-255)"=0, "Trigger Polarity"="", "External Trigger Mode"="", "Scan Speed"="", "External Trigger Source"="", "Scan Mode"="", "Super Pixel Binning\n(if enabled in Scan Mode)"="", "Camera Sub-array acquisition region\n(if enabled in scan mode)"={"Left"=0, "Top"=0, "Width"=0, "Height"=0}, "Use camera?"=FALSE, "# image buffers"=0, "Regions of Interest (Left, Top, Right, Bottom)"=[], "Background Regions (Left, Top, Right, Bottom)"=[], "shots per measurement"=0, "Photoelectron Scaling"=0.0, "Low Light\nSensitivity"="", "Save as TIF?"=FALSE, "Save as Raw .dat?"=FALSE, "Cooling"="", "Fan"=""}, "Counter Settings"={"Enable Counters"=FALSE, "Array of Counter Settings"=[], "#Bins to drop"=0, "Total Counts Active Bins"=[], "Histogram"={"Active Bins (Bin i:j)"=[], "Histogram?"=FALSE, "Accumulate?"=FALSE}}, "Filter Cluster"={"Counter Filter thresholds"=[], "Data Filters\nROI Minimum Thresholds"=[]}, "Analog Output Parameters"={"Enable Analog Out?"=FALSE, "Physical Channel"="", "Minimum Value"=0.0, "Maximum Value"=0.0, "Samples per second"="", "Total AO Time (seconds)"="", "Analog Output Equations for each Channel"=[], "Start Trigger"={"Wait for start trigger?"=FALSE, "source"="", "edge"=0}, "AO Channel List"=[]}, "Notes"="", "HP83623A Generator Settings Array"=[], "Iteration Graph Settings"={"Plot Regions"="", "Plot Shots"=""}, "PI Piezo Settings"={"Enable"=FALSE, "Array of Piezo Controllers"=[]}, "Andor settings"={"Andor Path"=path "", "Copy any Andor files"=FALSE, "Wait time before copying Andor files (ms)"=0}, "Measurement Chart Settings"={"Which regions to plot (comma separated)"="", "Which shot to plot"=0}, "HP8662A Synthesized Signal Generator Array"=[], "HP83712B Synthesized CW Generator Array"=[], "TTL input"={"Enable"=FALSE, "lines"=""}, "Luca Settings"={"Active Pixels (Left,Right,Top,Bottom)"=[], "Pixel Binning"="", "Use camera?"=FALSE, "Regions of Interest (Left, Top, Right, Bottom)"=[], "Background Regions (Left, Top, Right, Bottom)"=[], "Photoelectron Scaling"=0.0, "Save as TIF"=FALSE, "Save as Raw .dat"=FALSE, "Acquisition Mode"="", "Gain Mode"="", "Trigger Mode"="", "Fan Mode"="", "Advanced EMgain"=FALSE, "EMCCD Gain (0-200/1000)"=0, "Exposure (s)"=0.0, "#Kinetics"=0, "Hbin"=0, "Vbin"=0, "#H"=0, "#V"=0, "BG Subtraction"=FALSE}, "AFG3102 Frequency Control (kHz only)"={"Enable"=FALSE, "Description"="", "GPIB channel #"=0, "Frequency (MHz)"="", "Power (dBm)"=""}, "Aerotech Settings"={"Enable"=FALSE, "DGLOBAL Array"=[], "DGlobal_Update"=FALSE, "IGLOBAL Array"=[], "IGlobal_Update"=FALSE}, "CONEX-CC Settings"={"Enabled?"=FALSE, "Set Position"="", "Velocity (mm/s)"=0.0, "ModVel?"=FALSE}}  # all settings
        n14 = event-data() -> ()  [unwired: 1 in, 5 out]
        n15 = local read "Variable Settings"() -> (w28:T2)
        n16 = local read "DDS Settings"() -> (w24:T3)
        n17 = Bundle By Name(cluster=w29, "Variable Settings"=w28, "DDS Settings"=w24) -> (w27:T20)
        n18 = call "manual_save_settings.vi"("error in"=w26, "all settings"=w27) -> ("error out"=w25:errorcluster)  [unwired: 9 in]
      }
      event "DDS Actions.Load DDS": Value Change {
        n19 = event-data() -> ()  [unwired: 1 in, 5 out]
        n20 = local read "Variable Settings"() -> (w38:T2)
        n21 = local read "DDS Settings"() -> (w32:T3)
        n22 = call "get_variable_start_values.vi"("error in (no error)"=w31, "Variable Settings"=w38) -> ("error out"=w30:errorcluster, "all variable names"=w36:string[], "all variable values (min or calculated)"=w37:dbl[])  [unwired: 6 in, 1 out]
        n23 = call "DDS update.vi"("error in (no error)"=w30, "Variable Names"=w36, "Variable Values"=w37, "DDS Settings"=w32) -> ("error out"=w35:errorcluster)  [unwired: 7 in]
        n24 = property on="Load DDS" class="Bool (strict)"(error in=w35, "Value"=FALSE ("Load DDS")) -> (error out=w34:errorcluster)  [unwired: 1 in, 1 out]
      }
      event "Check DDS": Value Change {
        n25 = event-data() -> ()  [unwired: 1 in, 5 out]
        n26 = local read "DDS Settings"() -> (w40:T3)
        n27 = call "DDS_Check_Box.vi"("error in (no error)"=w45, "box #"="box #", "DDS Settings"=w40) -> ("error out"=w44:errorcluster, "CFR3"=→"CFR3":u8[][], "CFR2"=→"CFR2":u8[][], "CFR1"=→"CFR1":u8[][])  [unwired: 5 in]
      }
      event "Variable Actions.Load Independents": Value Change {
        n28 = event-data() -> ()  [unwired: 1 in, 5 out]
        n29 = call-poly <vilib>:"Read From Spreadsheet File.vi"() -> ("all rows"=w46:string[][])  [unwired: 7 in, 4 out]
        n30 = Delete From Array "Remove Header"(array=w46, length=1, index (row)=0 ("index")) -> (array with subset deleted=w47:string[][])  [unwired: 1 in, 1 out]
        n31 = for {
          shift-right: [w64] -> w52
          shift-left: w50 -> [w64]
          tunnel: w47 -> [w70] mode=indexing
          tunnel: [w72] -> w51 mode=indexing
          n32 = Index Array(array=w70, index #1=0 ("index"), index #2=1 ("index"), index #3=2 ("index"), index #4=3 ("index"), index #5=4 ("index")) -> (element #1=w63:string, element #2=w62:string, element #3=w61:string, element #4=w59:string, element #5=w57:string)
          n33 = Fract/Exp String To Number(string=w61) -> (number=w60:dbl)  [unwired: 3 in, 1 out]
          n34 = Fract/Exp String To Number(string=w59) -> (number=w58:dbl)  [unwired: 3 in, 1 out]
          n35 = Decimal String To Number(string=w57) -> (number=w56:i32)  [unwired: 2 in, 1 out]
          n36 = Bundle By Name(cluster=T18 {"Description"="", "Name (a,a0...a9)"="", "min"=0.0, "max"=0.0, "# steps"=0} ("Cluster"), "Description"=w63, "Name (a,a0...a9)"=w62, "min"=w60, "max"=w58, "# steps"=w56) -> (w72:T18)
        }
        n37 = property on="Independent Variables" class="Arr (strict)"(error in=w52, "Value"=w51) -> (error out=w53:errorcluster)  [unwired: 1 in, 1 out]
        n38 = property on="Load Independents" class="Bool (strict)"(error in=w53, "Value"=FALSE) -> (error out=w55:errorcluster)  [unwired: 1 in, 1 out]
      }
      event "Variable Actions.Load Dependents": Value Change {
        n39 = event-data() -> ()  [unwired: 1 in, 5 out]
        n40 = call-poly <vilib>:"Read From Spreadsheet File.vi"() -> ("all rows"=w74:string[][])  [unwired: 7 in, 4 out]
        n41 = Delete From Array "Remove Header"(array=w74, length=1, index (row)=0 ("index")) -> (array with subset deleted=w73:string[][])  [unwired: 1 in, 1 out]
        n42 = for {
          shift-right: [w88] -> w78
          shift-left: w80 -> [w88]
          tunnel: [w95] -> w79 mode=indexing
          tunnel: w73 -> [w93] mode=indexing
          n43 = Index Array(array=w93, index #1=0 ("index"), index #2=1 ("index"), index #3=2 ("index"), index #4=3 ("index")) -> (element #1=w87:string, element #2=w86:string, element #3=w85:string, element #4=w84:string)
          n44 = Fract/Exp String To Number(string=w84) -> (number=w83:dbl)  [unwired: 3 in, 1 out]
          n45 = Bundle By Name(cluster=T19 {"Description"="", "Name (a,a0...a9)"="", "Equation"="", "Result"=0.0} ("Cluster"), "Description"=w87, "Name (a,a0...a9)"=w86, "Equation"=w85, "Result"=w83) -> (w95:T19)
        }
        n46 = property on="Dependent Variables" class="Arr (strict)"(error in=w78, "Value"=w79) -> (error out=w77:errorcluster)  [unwired: 1 in, 1 out]
        n47 = property on="Load Dependents" class="Bool (strict)"(error in=w77, "Value"=FALSE) -> (error out=w82:errorcluster)  [unwired: 1 in, 1 out]
      }
      event "Variable Actions.Save Independents": Value Change {
        n48 = event-data() -> ()  [unwired: 1 in, 5 out]
        n49 = property on="Independent Variables" class="Arr (strict)"(error in=w99) -> (error out=w97:errorcluster, "Value"=w98:T45)  [unwired: 1 in, 1 out]
        n50 = call "save_variables_table.vi"("error in"=w97, "Variable Settings.Variables"=w98) -> ("error out"=w96:errorcluster)  [unwired: 9 in]
        n51 = property on="Return button to the unclicked position" class="Bool (strict)"(error in=w96, "Value"=FALSE) -> (error out=w100:errorcluster)  [unwired: 1 in, 1 out]
      }
      event "Variable Actions.Save Dependents": Value Change {
        n52 = event-data() -> ()  [unwired: 1 in, 5 out]
        n53 = property on="Dependent Variables" class="Arr (strict)"(error in=w105) -> (error out=w103:errorcluster, "Value"=w104:T46)  [unwired: 1 in, 1 out]
        n54 = call "save_parameters_table.vi"("error in"=w103, "Parameters"=w104) -> ("error out"=w102:errorcluster)  [unwired: 9 in]
        n55 = property on="Save Dependents" class="Bool (strict)"(error in=w102, "Value"=FALSE) -> (error out=w107:errorcluster)  [unwired: 1 in, 1 out]
      }
      event "Variable Actions.Clear Log": Value Change {
        n56 = event-data() -> ()  [unwired: 1 in, 5 out]
        n57 = call "clear_log.vi"("error in"=w109) -> ("error out"=w108:errorcluster)  [unwired: 10 in]
        n58 = property on="Clear Log" class="Bool (strict)"(error in=w108, "Value"=FALSE) -> (error out=w110:errorcluster)  [unwired: 1 in, 1 out]
      }
      event "Variable Actions.Evaluate Dependents": Value Change {
        n59 = event-data() -> ()  [unwired: 1 in, 5 out]
        n60 = local read "Variable Settings"() -> (w116:T2)
        n61 = call "get_variable_start_values.vi"("error in (no error)"=w115, "Variable Settings"=w116) -> ("error out"=w112:errorcluster, "dependent variable results"=w114:dbl[])  [unwired: 6 in, 2 out]
        n62 = property on="Dependent Variables" class="Arr (strict)"(error in=w112) -> (error out=w113:errorcluster, "Value"=w119:T46)  [unwired: 1 in, 1 out]
        n63 = for {
          tunnel: w114 -> [w124] mode=indexing
          tunnel: [w123] -> w118 mode=indexing
          tunnel: w119 -> [w122] mode=indexing
          n64 = Bundle By Name(cluster=w122, "Result"=w124) -> (w123:T19)
        }
        n65 = property on="Dependent Variables" class="Arr (strict)"(error in=w113, "Value"=w118) -> (error out=w117:errorcluster)  [unwired: 1 in, 1 out]
        n66 = property on="Evaluate Dependents" class="Bool (strict)"(error in=w117, "Value"=FALSE) -> (error out=w121:errorcluster)  [unwired: 1 in, 1 out]
      }
      event "DDS Actions.Initialize DDS Boxes": Value Change {
        n67 = event-data() -> ()  [unwired: 1 in, 5 out]
        n68 = local read "DDS Settings"() -> (w125:T3)
        n69 = Unbundle By Name(w125) -> ("Enable DDS"=w126:bool)
        n70 = case shown="True" w126 {
          tunnel: w130 -> [w131 w133]
          tunnel: [w131 w139] -> w128
          tunnel: w125 -> [_ w134]
          frame False {
          }
          frame True {
            n71 = local read "Variable Settings"() -> (w135:T2)
            n72 = call "get_variable_start_values.vi"("error in (no error)"=w133, "Variable Settings"=w135) -> ("error out"=w132:errorcluster, "all variable names"=w137:string[], "all variable values (min or calculated)"=w136:dbl[])  [unwired: 6 in, 1 out]
            n73 = call "DDS Startup.vi"("error in (no error)"=w132, "Variable Names"=w137, "Variable Values"=w136, "DDS Settings"=w134) -> ("error out"=w140:errorcluster)  [unwired: 7 in]
            n74 = property on="DDS Initialized" class="Bool (strict)"(error in=w140, "Value"=TRUE ("DDS Initialized")) -> (error out=w139:errorcluster)  [unwired: 1 in, 1 out]
          }
        }
        n75 = property on="Initialize DDS Boxes" class="Bool (strict)"(error in=w128, "Value"=FALSE ("DDS Initialized")) -> (error out=w127:errorcluster)  [unwired: 1 in, 1 out]
      }
      event "Quit Program": Value Change {
        n76 = event-data() -> ()  [unwired: 1 in, 5 out]
      }
    }
    n77 = call "handle_errors.vi"("error in (no error)"=w11) -> ("error out"=w9:errorcluster, "Stop"=w8:bool)  [unwired: 9 in]
    n78 = Or(x=w10, y=w8) -> (x .or. y?=w12:bool)
  }
  n79 = local read "DDS Settings"() -> (w4:T3)
  n80 = call "DDS_Close_Multiple_Boxes.vi"("error in (no error)"=w5, "DDS Settings"=w4) -> ("error out"=w3:errorcluster)  [unwired: 9 in]
  n81 = call <vilib>:"Simple Error Handler.vi"("type of dialog (OK msg:1)"=w6, "error in (no error)"=w3) -> ()  [unwired: 3 in, 5 out]
